vi "Demo User Notification and Status.vi"(8 "error in (no error)":errorcluster) -> (0 "error out":errorcluster)   [LabVIEW 2011]
uses:
  VIremote.llb/VIremoteEvent.ctl
  VIremote.llb/VIremoteStatus.ctl
  VIremote.llb/VIremoteFunction.ctl
  VIremote.llb/VIremotePopup.ctl
panel:
  in  "precision\nfor DBL":i16=2
  in  "all status":bool
  in  "Ring of status values":u16(ring) caption="Tilt to update" items=["Connected BOOL (True)", "Number of connections DBL (1.00)", "VIremoteController ver. (2.0)", "VIremote ver. DBL (2.00)", "Screen width DBL (320.00)", "Screen height DBL (480.00)", "Current navigation bar height DBL (0.00)", "Current UI orientation (3.00)", "Background supported BOOL (True)", "Background state BOOL (False)", "Device UI idiom (0=phone,1=iPad) DBL (0.00)", "Device name (iPhone Simulator)", "Device unique id (72516E35-C4A1-5474-AB87-7FE2C182CDC0)", "Device system ver. (5.0)", "Device model (iPhone Simulator)", "Device HW model (x86_64)"]
  in  "Status items (hidden type def)":T1
  in  "Message to be sent 1 second after VIremote enters background":string="Your LabVIEW VI needs your attention!"
  out "VIremoteEvent":T2=enum."Connection Closed"
  # "If you have a multitasking capable device (3GS and later) you can send a notification to the user when VIremote is running in the background. If it  is in the foreground nothing will happen.\n\nTo see this in action just press the home button."
  # "This button will populate a ring control with data from VIremoteStatus.vi and then set its KeyFocus to True. Which will cause the ring control to be displayed on the device. The ring is hidden under the button so that the arrow on the iPad popover wil point at the button.\n\nWith VIremoteStatus.vi you get info about VIremoteController and the current device."
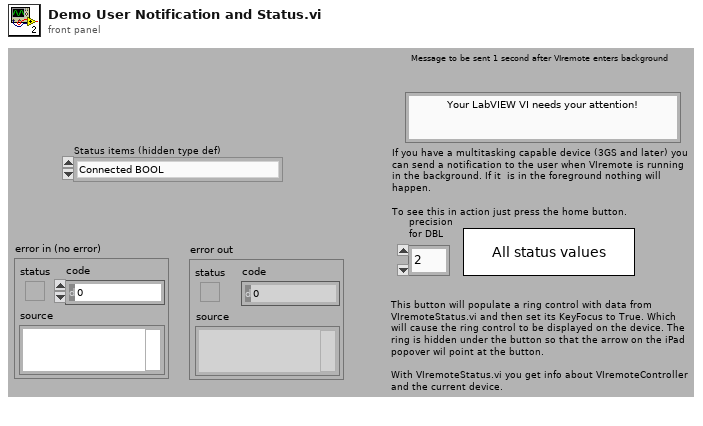
[diagram p1: front panel]
types:
  T1 = typedef "VIremoteStatus.ctl" = enum16{"Connected BOOL", "Number of connections DBL", "VIremoteController ver.", "VIremote ver. DBL", "Screen width DBL", "Screen height DBL", "Current navigation bar height DBL", "Current UI orientation", "Background supported BOOL", "Background state BOOL", "Device UI idiom (0=phone,1=iPad) DBL", "Device name", "Device unique id", "Device system ver.", "Device model", "Device HW model"}
  T2 = typedef "VIremoteEvent.ctl" = enum16{"No Event", "Connection Closed", "Navigate Back", "Enter Background", "Enter Foreground", "Portrait", "Portrait Upside Down", "Landscape Left", "Landscape Right"}
  T3 = typedef "VIremoteFunction.ctl" = enum16{"Do nothing", "Stop controller", "Close this connection", "Show info panel", "Set VI to control", "Set Accelerometer freq (Hz)", "Show Alert message", "Start Sound Input", "Stop Sound Input", "Set Volume (0-100)", "Set sound output Speaker", "Set sound output Receiver", "Play Sound", "Repeat Sound", "Stop Sound", "Pause Sound", "Resume Sound", "Set panel width of caller (320 or 480)", "Set Panel Size to Portrait", "Set Panel Size to Landscape", "Set Panel Size as Current Orientation", "Allow all UI Orientations", "Send user notification", "Disable Scrolling", "Normal Scrolling", "Page Scrolling", "Set Scroll Offset", "Page Indicator Position"}
  T4 = typedef "VIremotePopup.ctl" = enum16{"Show Popup", "Update popup if shown", "Get control refnum for shown popup"}
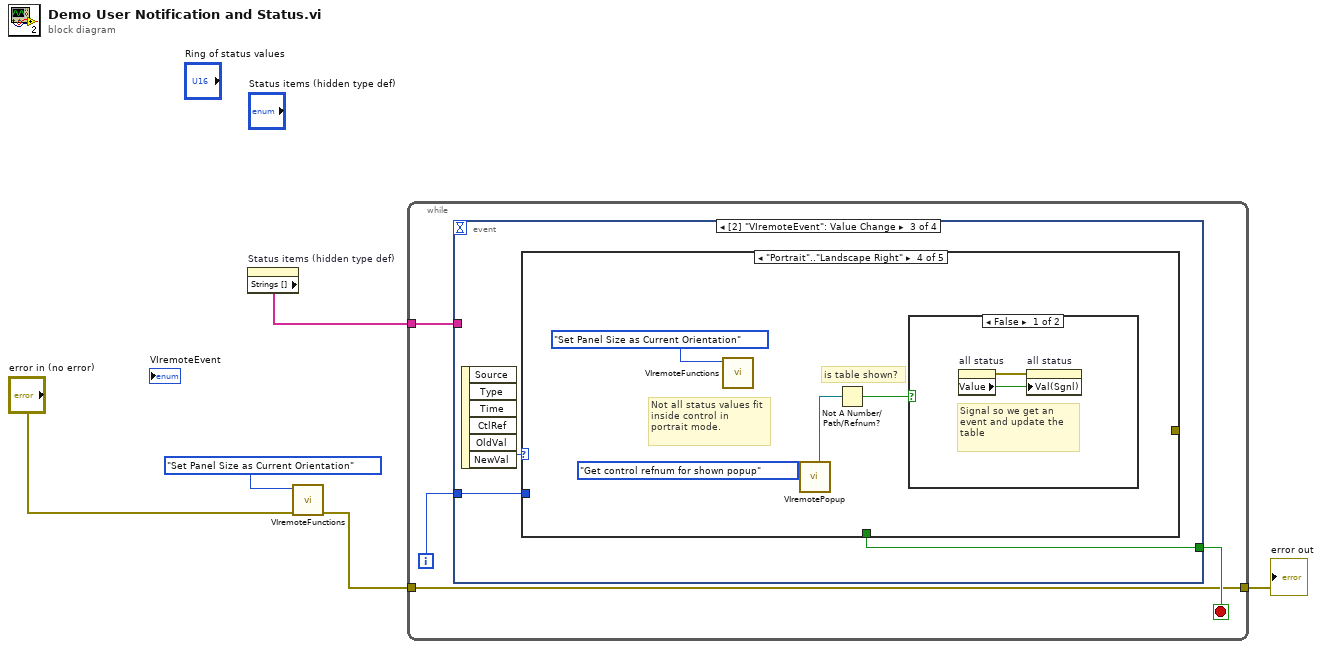
[diagram p0: block diagram]
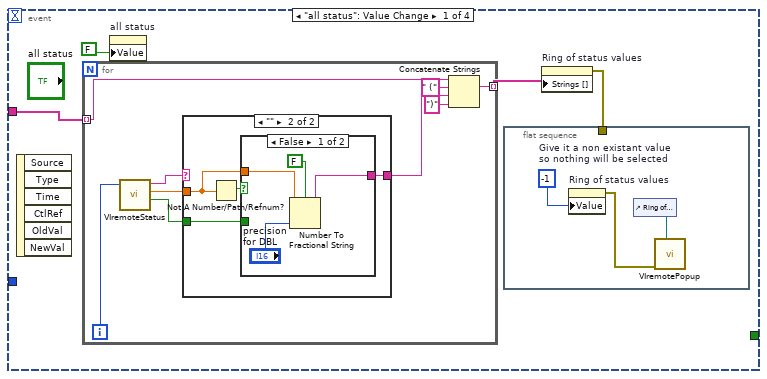
[diagram p2: hidden frame]
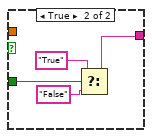
[diagram p4: hidden frame]
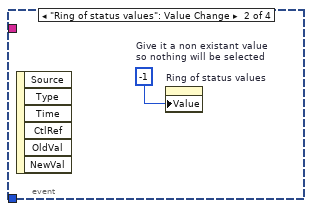
[diagram p5: hidden frame]
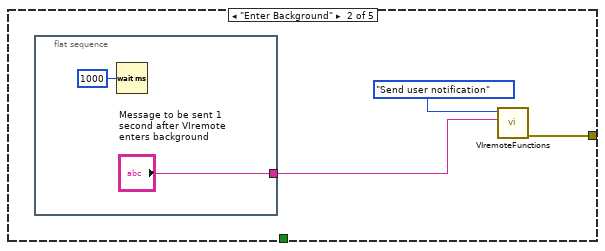
[diagram p7: hidden frame]
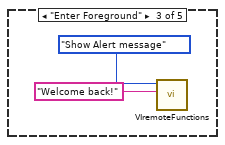
[diagram p8: hidden frame]
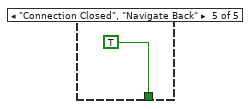
[diagram p10: hidden frame]
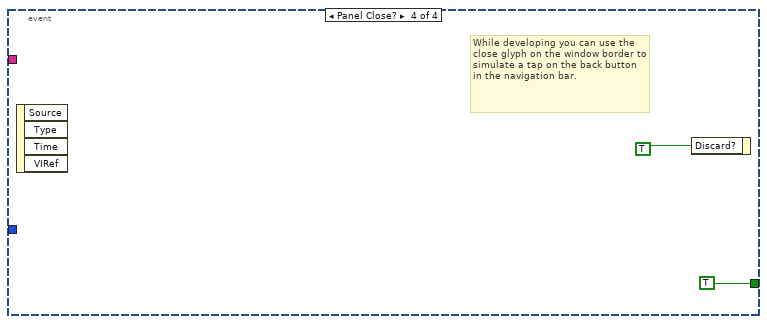
[diagram p11: hidden frame]
diagram:
  n1 = property on="Status items (hidden type def)" class="Enum (strict)"() -> ("Strings []"=w3:string[])  [unwired: 2 in, 2 out]
  n2 = call "VIremoteFunctions.vi"("error in (no error)"="error in (no error)", "Function"=VIremoteFunction."Set Panel Size as Current Orientation") -> ("error out"=w1:errorcluster)  [unwired: 4 in, 5 out]
  n3 = while {
    tunnel: w3 -> [w7]
    tunnel: [w6] -> w2
    tunnel: w1 -> [w6]
    i -> [w8]
    stop <- w9 stop-if-true
    n4 = event shown="[2] \"VIremoteEvent\": Value Change" {
      selector: _ -> [_ _ _ _]
      dyn-events: _ -> [_ _ _ _]
      timeout: _ -> [_ _ _ _]
      tunnel: [_ _ w42 TRUE ("Discard?")] -> w9
      tunnel: w8 -> [_ _ w40 _]
      tunnel: w7 -> [w13 _ _ _]
      event "all status": Value Change {
        n5 = event-data() -> ()  [unwired: 7 out]
        n6 = for {
          tunnel: w13 -> [w21] mode=indexing
          tunnel: [w17] -> w12 mode=indexing
          i -> [w22]
          n7 = call "VIremoteStatus.vi"("Status item"=w22) -> ("Bool"=w23:bool, "DBL"=w24:dbl, "String"=w25:string)  [unwired: 2 in, 6 out]
          n8 = case shown="\"\"" w25 {
            selector: w25 -> [w26 _]
            tunnel: [w26 w28] -> w20
            tunnel: w24 -> [_ w27]
            tunnel: w23 -> [_ w29]
            frame Default {
            }
            frame "" {
              n9 = Not A Number/Path/Refnum?(number/path/refnum=w27) -> (NaN/Path/Refnum?=w30:bool)
              n10 = case shown="False" w30 {
                tunnel: w29 -> [_ w38]
                tunnel: [w33 w37] -> w28
                tunnel: w27 -> [w34 _]
                frame False {
                  n11 = Number To Fractional String(use system decimal point (T)=FALSE, number=w34, precision (6)="precision\nfor DBL") -> (F-format string=w33:string)  [unwired: 1 out]
                }
                frame True {
                  n12 = Select(t="True", s=w38, f="False") -> (s? t:f=w37:string)
                }
              }
            }
          }
          n13 = Concatenate Strings(w21, " (" ("string"), w20, ")" ("string")) -> (w17:string)
        }
        n14 = property on="all status" class="Bool (strict)"("Value"=FALSE) -> ()  [unwired: 2 in, 2 out]
        n15 = flat-sequence {
          tunnel: w11 -> [_]
          frame #0 {
            w16 = -1  # Give it a non existant value so nothing will be selected
            n16 = property on="Ring of status values" class="Ring (strict)"("Value"=w16) -> (error out=w14:errorcluster)  [unwired: 2 in, 1 out]
            n17 = control-ref of="Ring of status values"() -> (w15:refnum<vi>)
            n18 = call "VIremotePopup.vi"("Control Refnum"=w15, "error in (no error)"=w14) -> ()  [unwired: 10 out]
          }
        }
        n19 = property on="Ring of status values" class="Ring (strict)"("Strings []"=w12) -> (error out=w11:errorcluster)  [unwired: 2 in, 1 out]
      }
      event "Ring of status values": Value Change {
        w39 = -1  # Give it a non existant value so nothing will be selected
        n20 = event-data() -> ()  [unwired: 7 out]
        n21 = property on="Ring of status values" class="Ring (strict)"("Value"=w39) -> ()  [unwired: 2 in, 2 out]
      }
      event Value Change {
        n22 = event-data() -> ("NewVal"=w41:T2)  [unwired: 6 out]
        n23 = case shown="\"Portrait\"..\"Landscape Right\"" w41 {
          tunnel: [_ _ _ _ TRUE] -> w42
          tunnel: w40 -> [_ _ _ _ _]
          tunnel: [_ w43 _ _ _] -> _
          frame "No Event", Default {
          }
          frame "Enter Background" {
            n24 = flat-sequence {
              tunnel: ["Message to be sent 1 second after VIremote enters background"] -> w44
              frame #0 {
                n25 = Wait (ms)(milliseconds to wait=u32 1000) -> ()  [unwired: 1 out]
              }
            }
            n26 = call "VIremoteFunctions.vi"("String in"=w44, "Function"=VIremoteFunction."Send user notification") -> ("error out"=w43:errorcluster)  [unwired: 4 in, 5 out]
          }
          frame "Enter Foreground" {
            n27 = call "VIremoteFunctions.vi"("String in"="Welcome back!", "Function"=VIremoteFunction."Show Alert message") -> ()  [unwired: 4 in, 6 out]
          }
          frame "Portrait".."Landscape Right" {
            # "is table shown?"
            # "Not all status values fit inside control in portrait mode."
            n28 = call "VIremoteFunctions.vi"("Function"=VIremoteFunction."Set Panel Size as Current Orientation") -> ()  [unwired: 5 in, 6 out]
            n29 = call "VIremotePopup.vi"("Function (Show Popup)"=VIremotePopup."Get control refnum for shown popup" ("Function")) -> ("Control Refnum Out"=w52:refnum<vi>)  [unwired: 1 in, 9 out]
            n30 = Not A Number/Path/Refnum?(number/path/refnum=w52) -> (NaN/Path/Refnum?=w51:bool)
            n31 = case shown="False" w51 {
              frame False {
                # "Signal so we get an event and update the table"
                n32 = property on="all status" class="Bool (strict)"() -> (error out=w55:errorcluster, "Value"=w54:bool)  [unwired: 2 in, 1 out]
                n33 = property on="all status" class="Bool (strict)"(error in=w55, "Val(Sgnl)"=w54) -> ()  [unwired: 1 in, 2 out]
              }
              frame True {
              }
            }
          }
          frame "Connection Closed", "Navigate Back" {
          }
        }
      }
      event Panel Close? {
        # "While developing you can use the close glyph on the window border to simulate a tap on the back button in the navigation bar."
        n34 = event-data() -> ()  [unwired: 5 out]
        n35 = event-data("Discard?"=TRUE) -> ()  [unwired: 1 in, 1 out]
      }
    }
  }
  "error out" <- w2
